vi "fgv_statistics.vi"(7 "cmd":T2, 11 "statistics values":T1) -> (3 "statistics values out":T1)   [LabVIEW 2019]
uses:
  Ctrl/cmd_ini-RW.ctl
  Ctrl/statistics_val.ctl
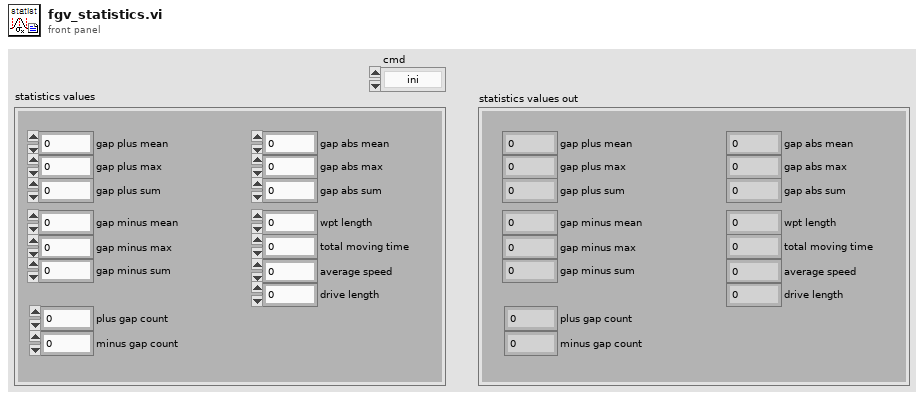
[diagram p1: front panel]
types:
  T1 = typedef "statistics_val.ctl" = cluster{"gap plus mean":dbl, "gap plus max":dbl, "gap plus sum":dbl, "gap minus mean":dbl, "gap minus max":dbl, "gap minus sum":dbl, "gap abs mean":dbl, "gap abs max":dbl, "gap abs sum":dbl, "wpt length":dbl, "total moving time":dbl, "average speed":dbl, "plus gap count":u64, "minus gap count":u64, "drive length":dbl}
  T2 = typedef "cmd_ini-RW.ctl" = enum16{"ini", "read", "write"}
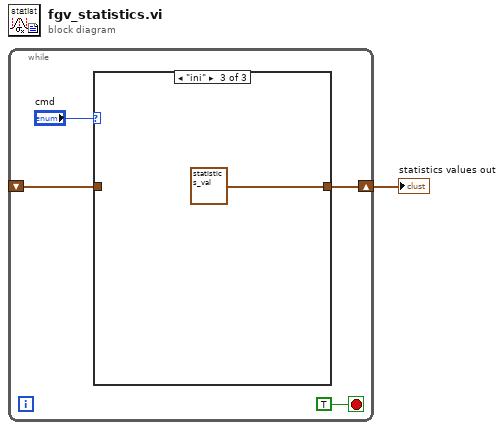
[diagram p0: block diagram]
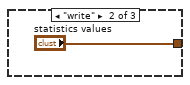
[diagram p3: hidden frame]
diagram:
  n1 = while {
    shift-right: [w3] -> w1
    shift-left: _ -> [w2]
    stop <- TRUE stop-if-true
    n2 = case shown="\"ini\"" "cmd" {
      tunnel: [w6 "statistics values" T1 {"gap plus mean"=0.0, "gap plus max"=0.0, "gap plus sum"=0.0, "gap minus mean"=0.0, "gap minus max"=0.0, "gap minus sum"=0.0, "gap abs mean"=0.0, "gap abs max"=0.0, "gap abs sum"=0.0, "wpt length"=0.0, "total moving time"=0.0, "average speed"=0.0, "plus gap count"=0, "minus gap count"=0, "drive length"=0.0} ("statistics values")] -> w3
      tunnel: w2 -> [w6 _ _]
      frame "read", Default {
      }
      frame "write" {
      }
      frame "ini" {
      }
    }
  }
  "statistics values out" <- w1
